vi "Get IP in Subnet.vi"(8 "error in (no error)":errorcluster, 10 "Address to Match":u32 format="%08x", 11 "Address to Match":string) -> (0 "error out":errorcluster, 2 "IPV4 Address":T1 {"Mask" format="%08x"; "Address" format="%08x"}, 3 "IPV4 Address":string)   [LabVIEW 2021, in "Networking_CIF_U.lvlib"]
uses:
  Networking_CIF_U.lvlib
  Typedef/Errors.ctl
  Typedef/IPV4 Address.ctl
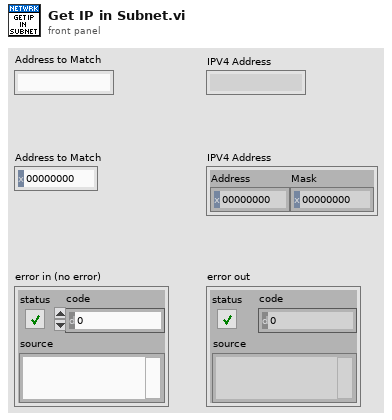
[diagram p1: front panel]
types:
  T1 = typedef "Networking_CIF_U.lvlib/IPV4 Address.ctl" = cluster{"Address":u32, "Mask":u32}
  T2 = typedef "Networking_CIF_U.lvlib/Errors.ctl" = enum16{"Invalid IP Address", "No Subnet Match Found", "Error Finding Port", "No Ping Response", "Nettools Needed"}
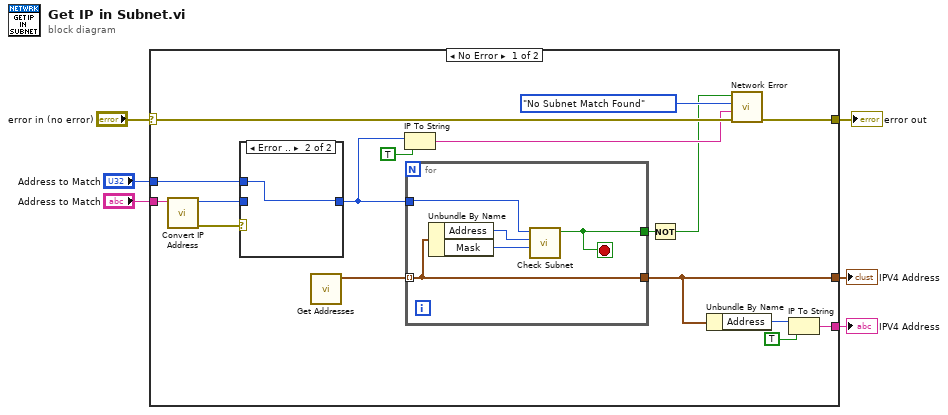
[diagram p0: block diagram]
diagram:
  n1 = case shown="No Error" "error in (no error)" {
    selector: "error in (no error)" -> [w12 w31]
    tunnel: "Address to Match" -> [w23 _]
    tunnel: "Address to Match" -> [w20 _]
    tunnel: [w16 _] -> w4
    tunnel: [w15 _] -> w3
    tunnel: [w13 w31] -> w2
    frame No Error {
      n2 = call "Convert IP Address.vi"("IP"=w23) -> ("error out"=w22:errorcluster, "net address"=w21:u32)  [unwired: 9 in]
      n3 = case shown="Error .." w22 {
        tunnel: w21 -> [w29 _]
        tunnel: [w29 w30] -> w10
        tunnel: w20 -> [_ w30]
        frame No Error {
        }
        frame Error {
        }
      }
      n4 = call "Get Addresses.vi"() -> ("IP Addresses"=w19:T1[])  [unwired: 10 in, 1 out]
      n5 = IP To String(1:TRUE ("dot notation? (F)"), 2:w10) -> (0:w9:string)
      n6 = for {
        tunnel: w19 -> [w25] mode=indexing
        tunnel: w10 -> [w28]
        tunnel: [w25] -> w16
        tunnel: [w24] -> w14
        stop <- w24 stop-if-true
        n7 = Unbundle By Name(w25) -> ("Address"=w27:u32, "Mask"=w26:u32)
        n8 = call "Check Subnet.vi"("Mask"=w26, "Address 2"=w27, "Address 1"=w28) -> ("In Subnet"=w24:bool)  [unwired: 8 in]
      }
      n9 = Not(x=w14) -> (.not. x?=w7:bool)
      n10 = Unbundle By Name(w16) -> ("Address"=w18:u32)
      n11 = call "Network Error.vi"("error in (no error)"=w12, "String to Append"=w9, "Error"=Errors."No Subnet Match Found", "Insert Error"=w7) -> ("error out"=w13:errorcluster)  [unwired: 7 in]
      n12 = IP To String(1:TRUE ("dot notation? (F)"), 2:w18) -> (0:w15:string)
    }
    frame Error {
    }
  }
  "IPV4 Address" <- w4
  "IPV4 Address" <- w3
  "error out" <- w2
